vi "Create simple HTML Documentation for this VI.vi"(11 "error in (no error)":errorcluster) -> (15 "error out":errorcluster)   [LabVIEW 2012]
doc: "This command will create simple VI documentation in HTML format similar to built-in LabVIEW 'Print VI' option."
uses:
  <vilib>/Platform/browser.llb/Open URL in Default Browser (path).vi
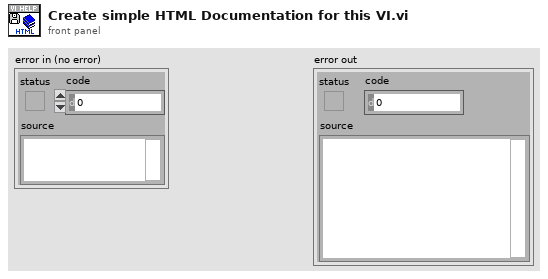
[diagram p1: front panel]
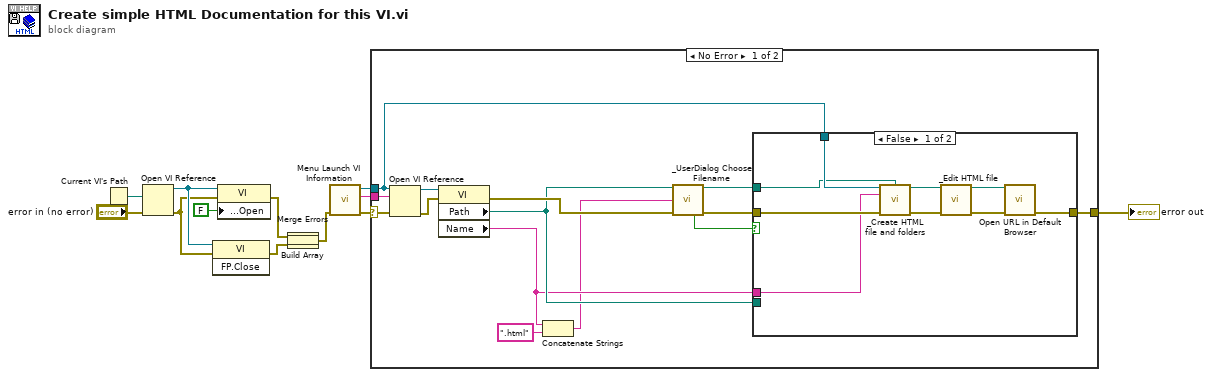
[diagram p0: block diagram]
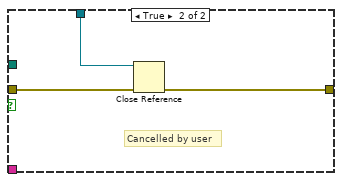
[diagram p2: hidden frame]
diagram:
  n1 = Current VI's Path() -> (path=w9:path)
  n2 = Open VI Reference(vi path=w9, error in (no error)="error in (no error)") -> (vi reference=w6:refnum<vi>, error out=w5:errorcluster)  [unwired: 4 in]
  n3 = invoke class="VI" method="FP.Close"(reference=w6, error in=w5) -> (error out=w3:errorcluster)  [unwired: 1 in, 2 out]
  n4 = property class="VI"(reference=w6, error in=w5, "Front Panel.Open"=FALSE ("Front Panel Window:Open")) -> (error out=w4:errorcluster)  [unwired: 1 out]
  n5 = Build Array(w4, w3) -> (w1:errorcluster[])
  n6 = Merge Errors(w1) -> (w2:errorcluster)
  n7 = call <vilib>:"Menu Launch VI Information.vi"("error in (no error)"=w2) -> ("error out"=w11:errorcluster, "Menu Launch:VI"=w12:string, "Menu Launch:App"=w13:refnum<vi>)  [unwired: 8 in]
  n8 = case shown="No Error" w11 {
    selector: w11 -> [w25 w40]
    tunnel: [w27 w40] -> w10
    tunnel: w13 -> [w22 _]
    tunnel: w12 -> [w20 _]
    frame No Error {
      n9 = Open VI Reference(application reference (local)=w22, vi path=w20, error in (no error)=w25) -> (vi reference=w26:refnum<vi>, error out=w24:errorcluster)  [unwired: 3 in]
      n10 = property class="VI"(reference=w26, error in=w24) -> (error out=w23:errorcluster, "Path"=w18:path, "Name"=w17:string)  [unwired: 1 out]
      n11 = Concatenate Strings(w17, ".html" ("string")) -> (w16:string)
      n12 = call "_UserDialog Choose Filename.vi"("VI Default Path"=w18, "Default file name"=w16, "error in (no error)"=w23) -> ("HTML File Path"=w19:path, "Cancelled by User?"=w14:bool, "error out"=w21:errorcluster)  [unwired: 8 in, 2 out]
      n13 = case shown="False" w14 {
        tunnel: [w29 w37] -> w27
        tunnel: w22 -> [w34 w39]
        tunnel: w21 -> [w33 w38]
        tunnel: w19 -> [w32 _]
        tunnel: w18 -> [_ _]
        tunnel: w17 -> [w31 _]
        frame False {
          n14 = call "_Create HTML file and folders.vi"("Menu Launch:App"=w34, "HTML File Path"=w32, "Menu Launch:VI"=w31, "error in (no error)"=w33) -> ("HTML FIle Path out"=w35:path, "error out"=w36:errorcluster)  [unwired: 10 in]
          n15 = call "_Edit HTML file.vi"("HTML File Path"=w35, "error in"=w36) -> ("HTML File Path out"=w28:path, "error out"=w30:errorcluster)  [unwired: 12 in]
          n16 = call-poly <vilib>:"Open URL in Default Browser.vi"("error in (no error)"=w30, "path"=w28) -> ("error out"=w29:errorcluster)  [unwired: 4 in, 1 out]
        }
        frame True {
          # "Cancelled by user"
          n17 = Close Reference(reference=w39, error in (no error)=w38) -> (error out=w37:errorcluster)
        }
      }
    }
    frame Error {
    }
  }
  "error out" <- w10
